vi "robot_alignment.vi"(4 "Direction":i8) -> ()   [LabVIEW 2012]
uses:
  Global_var.vi
  <userlib>/dhd_sdk7/dhd_sdk7.lvlib
panel:
  in  "stop":bool
  out "Target":dbl[](array[numeric])
  # "Performing robot alignment test. \nPress \"STOP\" button to quit."
  # "degree"
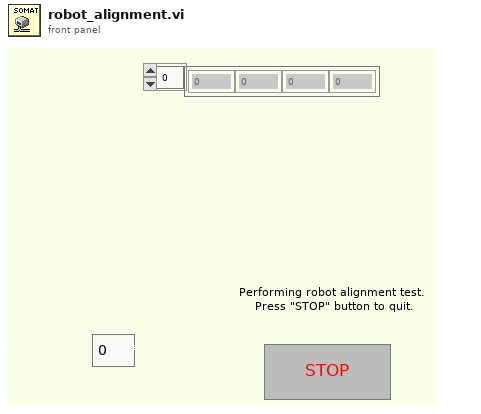
[diagram p1: front panel]
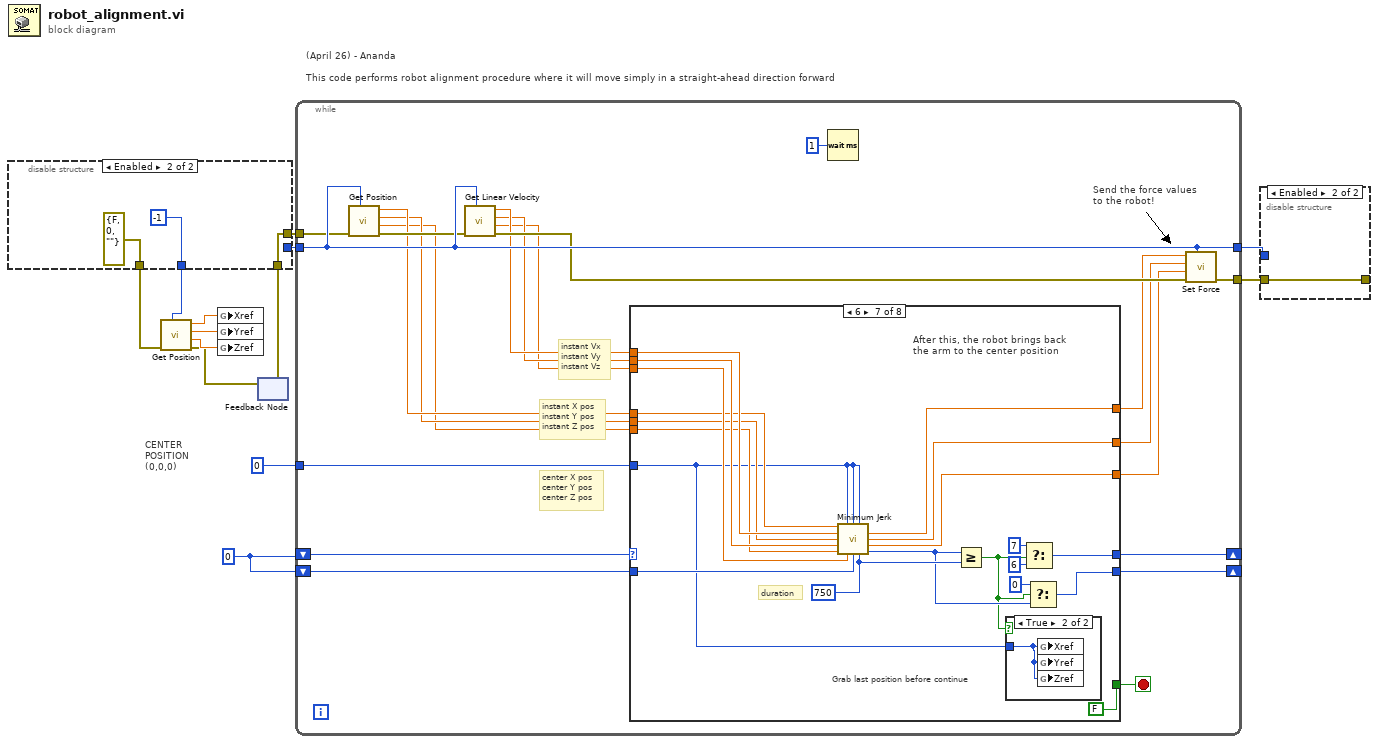
[diagram p0: block diagram]
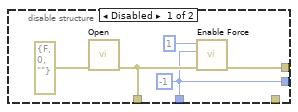
[diagram p2: hidden frame]
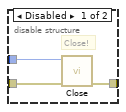
[diagram p3: hidden frame]
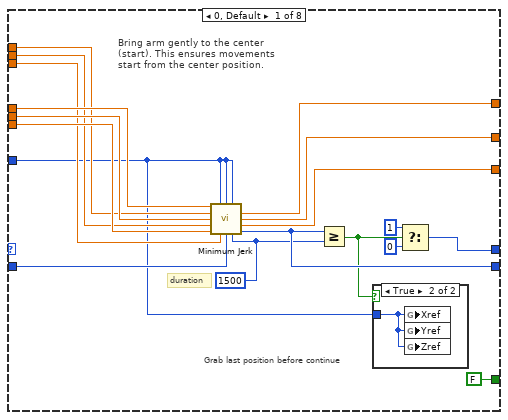
[diagram p4: hidden frame]
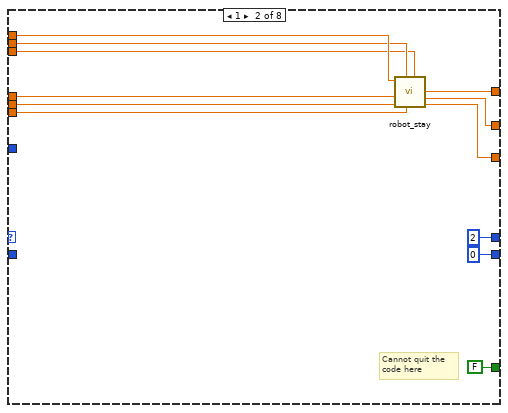
[diagram p6: hidden frame]
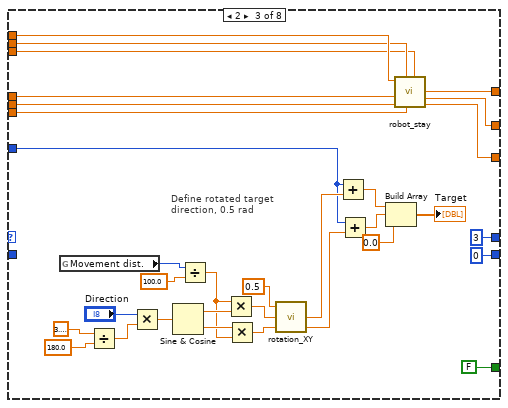
[diagram p7: hidden frame]
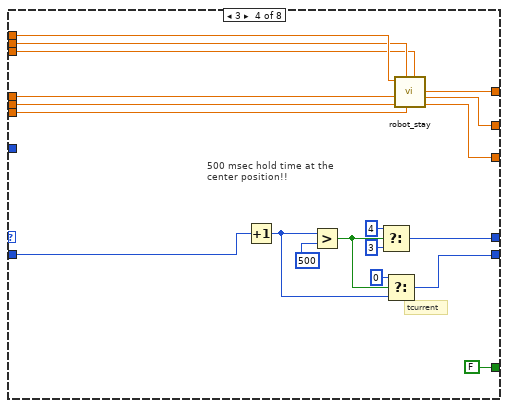
[diagram p8: hidden frame]
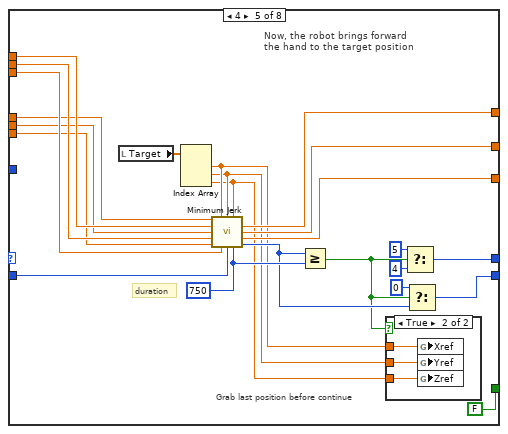
[diagram p9: hidden frame]
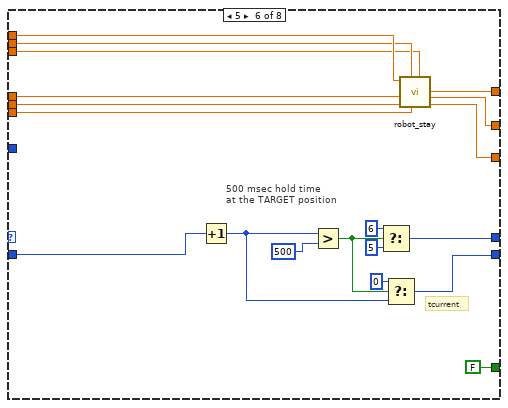
[diagram p11: hidden frame]
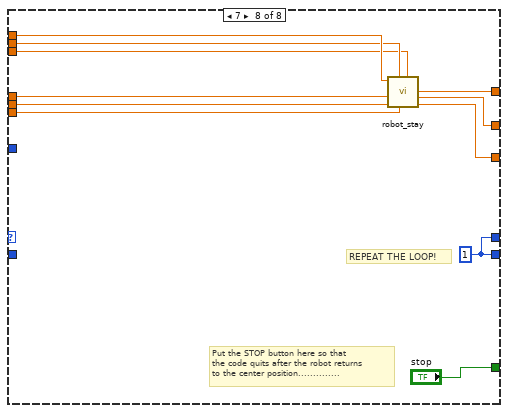
[diagram p13: hidden frame]
diagram:
  w10 = u16 0 ("ID")
  # "(April 26) - Ananda\n\nThis code performs robot alignment procedure where it will move simply in a straight-ahead direction forward"
  # "CENTER \nPOSITION\n(0,0,0)"
  n1 = feedback #1() -> (w1:errorcluster)  [unwired: 1 in]
  n2 = disable-structure shown="Enabled" {
    disable-tunnel: [w16 w19] -> w12
    disable-tunnel: [w14 _] -> w11
    disable-tunnel: [w15 errorcluster {"status"=FALSE, "code"=0, "source"=""} ("error out")] -> w4
    disable-tunnel: [w14 i8 -1 ("ID")] -> w3
    disable-tunnel: w1 -> [_ w19]
    frame Disabled {
      w14 = i8 -1 ("ID")
      n3 = call <userlib>:"Open.vi"("error in (no error)"=errorcluster {"status"=FALSE, "code"=0, "source"=""} ("error out")) -> ("error out"=w15:errorcluster)  [unwired: 9 in, 1 out]
      n4 = call <userlib>:"Enable Force.vi"("error in (no error)"=w15, "ID"=w14, "val"=u8 1) -> ("error out"=w16:errorcluster)  [unwired: 7 in, 1 out]
    }
    frame Enabled {
    }
  }
  n5 = call <userlib>:"Get Position.vi"("ID"=w3, "error in (no error)"=w4) -> ("error out"=w2:errorcluster, "pz out"=w5:dbl, "py out"=w6:dbl, "px out"=w7:dbl)  [unwired: 5 in, 1 out]
  n6 = global write "Global_var.vi" "Xref"(w7) -> ()
  n7 = global write "Global_var.vi" "Yref"(w6) -> ()
  n8 = global write "Global_var.vi" "Zref"(w5) -> ()
  n9 = feedback-in #1(w2) -> ()
  n10 = while {
    tunnel: w11 -> [w40]
    shift-right: [w42] -> _
    shift-left: w10 -> [w41]
    tunnel: [w40] -> w13
    tunnel: w12 -> [w39]
    shift-right: [w37] -> _
    shift-left: w10 -> [w38]
    tunnel: [w36] -> w9
    tunnel: u16 0 ("ID") -> [w24]
    stop <- w22 stop-if-true
    # "center X pos\ncenter Y pos\ncenter Z pos"
    # "Send the force values to the robot!"
    # "instant Vx\ninstant Vy\ninstant Vz"
    # "instant X pos\ninstant Y pos\ninstant Z pos"
    n11 = call <userlib>:"Get Position.vi"("ID"=w40, "error in (no error)"=w39) -> ("error out"=w35:errorcluster, "pz out"=w28:dbl, "py out"=w29:dbl, "px out"=w30:dbl)  [unwired: 5 in, 1 out]
    n12 = call <userlib>:"Get Linear Velocity.vi"("ID"=w40, "error in (no error)"=w35) -> ("error out"=w34:errorcluster, "vz out"=w25:dbl, "vy out"=w26:dbl, "vx out"=w27:dbl)  [unwired: 5 in, 1 out]
    n13 = case shown="6" w41 {
      tunnel: [w58 u8 2 ("ID") u8 3 ("ID") w124 w134 w166 w176 w201] -> w42
      tunnel: [w54 w66 w83 w115 w137 w154 w180 w194] -> w33
      tunnel: [w55 w65 w81 w114 w136 w153 w179 w193] -> w32
      tunnel: w38 -> [w52 _ _ w122 w138 w162 w177 _]
      tunnel: [w57 u32 0 ("ID") u32 0 ("ID") w123 w132 w164 w173 w201] -> w37
      tunnel: [w56 w64 w82 w113 w135 w152 w178 w192] -> w31
      tunnel: w30 -> [w51 w69 w86 w118 w141 w157 w183 w197]
      tunnel: w29 -> [w50 w68 w85 w117 w140 w156 w182 w196]
      tunnel: w28 -> [w49 w67 w84 w116 w139 w155 w181 w195]
      tunnel: w27 -> [w48 w72 w89 w121 w144 w160 w186 w200]
      tunnel: w26 -> [w47 w71 w88 w120 w143 w159 w185 w199]
      tunnel: w25 -> [w46 w70 w87 w119 w142 w158 w184 w198]
      tunnel: w24 -> [w44 _ w75 _ _ _ w172 _]
      tunnel: [FALSE ("stop") FALSE ("stop") FALSE ("stop") FALSE ("stop") FALSE ("stop") FALSE ("stop") FALSE ("stop") "stop"] -> w22
      frame 0, Default {
        w53 = u16 1500 ("duration")
        # "Grab last position before continue"
        # "Bring arm gently to the center\n(start). This ensures movements\nstart from the center position."
        # "duration"
        n14 = call "Minimum Jerk.vi"("X"=w51, "Xfinal"=w44, "Yfinal"=w44, "Zfinal"=w44, "Vx"=w48, "Y"=w50, "Vy"=w47, "Z"=w49, "Vz"=w46, "current_n"=w52, "duration"=w53) -> ("Fx"=w54:dbl, "Fy"=w55:dbl, "Fz"=w56:dbl, "n out"=w57:u16)  [unwired: 1 out]
        n15 = Greater Or Equal?(x=w57, y=w53) -> (x >= y?=w45:bool)
        n16 = case shown="True" w45 {
          tunnel: w44 -> [_ w61]
          frame False {
          }
          frame True {
            n17 = global write "Global_var.vi" "Xref"(w61) -> ()
            n18 = global write "Global_var.vi" "Yref"(w61) -> ()
            n19 = global write "Global_var.vi" "Zref"(w61) -> ()
          }
        }
        n20 = Select(t=u8 1 ("ID"), s=w45, f=u8 0) -> (s? t:f=w58:u8)
      }
      frame 1 {
        # "Cannot quit the\ncode here"
        n21 = call "robot_stay.vi"("Vz"=w70, "Z"=w67, "Vy"=w71, "Y"=w68, "X"=w69, "Vx"=w72) -> ("Fz"=w64:dbl, "Fy"=w65:dbl, "Fx"=w66:dbl)  [unwired: 3 in]
      }
      frame 2 {
        # "Define rotated target direction, 0.5 rad"
        n22 = global read "Global_var.vi" "Movement dist."() -> (w103:u8)
        n23 = Divide(x=3.141592653589793, y=180.0) -> (x/y=w78:dbl)
        n24 = Multiply(x="Direction", y=w78) -> (x*y=w76:dbl)
        n25 = Sine & Cosine(0:w76) -> (1:w104:dbl, 2:w105:dbl)
        n26 = Divide(x=w103, y=100.0) -> (x/y=w101:dbl)
        n27 = Multiply(x=w101, y=w104) -> (x*y=w99:dbl)
        n28 = Multiply(x=w105, y=w101) -> (x*y=w100:dbl)
        n29 = call "rotation_XY.vi"("y_pos"=w100, "x_pos"=w99, "angle"=0.5 ("theta")) -> ("rot_y"=w96:dbl, "rot_x"=w97:dbl)  [unwired: 1 in]
        n30 = Add(x=w75, y=w97) -> (x+y=w94:dbl)
        n31 = Add(x=w75, y=w96) -> (x+y=w93:dbl)
        n32 = Build Array(w94, w93, 0.0 ("element")) -> (→"Target":dbl[])
        n33 = call "robot_stay.vi"("Vz"=w87, "Z"=w84, "Vy"=w88, "Y"=w85, "X"=w86, "Vx"=w89) -> ("Fz"=w82:dbl, "Fy"=w81:dbl, "Fx"=w83:dbl)  [unwired: 3 in]
      }
      frame 3 {
        # "500 msec hold time at the center position!!"
        # "tcurrent"
        n34 = Increment(x=w122) -> (x+1=w107:u32)
        n35 = Greater?(x=w107, y=u32 500) -> (0:w108:bool)
        n36 = Select(t=u8 4 ("ID"), s=w108, f=u8 3) -> (s? t:f=w124:u8)
        n37 = Select(t=u8 0 ("ID"), s=w108, f=w107) -> (s? t:f=w123:u32)
        n38 = call "robot_stay.vi"("Vz"=w119, "Z"=w116, "Vy"=w120, "Y"=w117, "X"=w118, "Vx"=w121) -> ("Fz"=w113:dbl, "Fy"=w114:dbl, "Fx"=w115:dbl)  [unwired: 3 in]
      }
      frame 4 {
        w145 = u16 750 ("duration")
        # "Grab last position before continue"
        # "Now, the robot brings forward\nthe hand to the target position"
        # "duration"
        n39 = local read "Target"() -> (w130:dbl[])
        n40 = Index Array(array=w130) -> (element #1=w128:dbl, element #2=w127:dbl, element #3=w126:dbl)  [unwired: 3 in]
        n41 = call "Minimum Jerk.vi"("X"=w141, "Xfinal"=w128, "Yfinal"=w127, "Zfinal"=w126, "Vx"=w144, "Y"=w140, "Vy"=w143, "Z"=w139, "Vz"=w142, "current_n"=w138, "duration"=w145) -> ("Fx"=w137:dbl, "Fy"=w136:dbl, "Fz"=w135:dbl, "n out"=w131:u16)  [unwired: 1 out]
        n42 = Greater Or Equal?(x=w131, y=w145) -> (x >= y?=w129:bool)
        n43 = case shown="True" w129 {
          tunnel: w128 -> [_ w150]
          tunnel: w127 -> [_ w149]
          tunnel: w126 -> [_ w148]
          frame False {
          }
          frame True {
            n44 = global write "Global_var.vi" "Xref"(w150) -> ()
            n45 = global write "Global_var.vi" "Yref"(w149) -> ()
            n46 = global write "Global_var.vi" "Zref"(w148) -> ()
          }
        }
        n47 = Select(t=u8 5 ("ID"), s=w129, f=u8 4) -> (s? t:f=w134:u8)
        n48 = Select(t=u16 0, s=w129, f=w131) -> (s? t:f=w132:u16)
      }
      frame 5 {
        # "500 msec hold time\nat the TARGET position"
        # "tcurrent"
        n49 = Increment(x=w162) -> (x+1=w161:u32)
        n50 = Greater?(x=w161, y=u32 500) -> (0:w163:bool)
        n51 = Select(t=u8 6 ("ID"), s=w163, f=u8 5) -> (s? t:f=w166:u8)
        n52 = Select(t=u8 0 ("ID"), s=w163, f=w161) -> (s? t:f=w164:u32)
        n53 = call "robot_stay.vi"("Vz"=w158, "Z"=w155, "Vy"=w159, "Y"=w156, "X"=w157, "Vx"=w160) -> ("Fz"=w152:dbl, "Fy"=w153:dbl, "Fx"=w154:dbl)  [unwired: 3 in]
      }
      frame 6 {
        w187 = u16 750 ("duration")
        # "Grab last position before continue"
        # "After this, the robot brings back\nthe arm to the center position"
        # "duration"
        n54 = call "Minimum Jerk.vi"("X"=w183, "Xfinal"=w172, "Yfinal"=w172, "Zfinal"=w172, "Vx"=w186, "Y"=w182, "Vy"=w185, "Z"=w181, "Vz"=w184, "current_n"=w177, "duration"=w187) -> ("Fx"=w180:dbl, "Fy"=w179:dbl, "Fz"=w178:dbl, "n out"=w174:u16)  [unwired: 1 out]
        n55 = Greater Or Equal?(x=w174, y=w187) -> (x >= y?=w171:bool)
        n56 = case shown="True" w171 {
          tunnel: w172 -> [_ w190]
          frame False {
          }
          frame True {
            n57 = global write "Global_var.vi" "Xref"(w190) -> ()
            n58 = global write "Global_var.vi" "Yref"(w190) -> ()
            n59 = global write "Global_var.vi" "Zref"(w190) -> ()
          }
        }
        n60 = Select(t=u8 7 ("ID"), s=w171, f=u8 6) -> (s? t:f=w176:u8)
        n61 = Select(t=u16 0, s=w171, f=w174) -> (s? t:f=w173:u16)
      }
      frame 7 {
        w201 = u8 1 ("ID")
        # "Put the STOP button here so that\nthe code quits after the robot returns\nto the center position.............."
        # "REPEAT THE LOOP!"
        n62 = call "robot_stay.vi"("Vz"=w198, "Z"=w195, "Vy"=w199, "Y"=w196, "X"=w197, "Vx"=w200) -> ("Fz"=w192:dbl, "Fy"=w193:dbl, "Fx"=w194:dbl)  [unwired: 3 in]
      }
    }
    n63 = Wait (ms)(milliseconds to wait=u32 1) -> ()  [unwired: 1 out]
    n64 = call <userlib>:"Set Force.vi"("ID"=w40, "error in (no error)"=w34, "fz"=w31, "fy"=w32, "fx"=w33) -> ("error out"=w36:errorcluster)  [unwired: 5 in, 1 out]
  }
  n65 = disable-structure shown="Enabled" {
    disable-tunnel: w13 -> [w204 _]
    disable-tunnel: w9 -> [w203 w205]
    disable-tunnel: [w202 w205] -> _
    frame Disabled {
      # "Close!"
      n66 = call <userlib>:"Close.vi"("error in (no error)"=w203, "ID"=w204) -> ("error out"=w202:errorcluster)  [unwired: 8 in, 1 out]
    }
    frame Enabled {
    }
  }
